vi "Write Integer Result to Log.vi"(7 "Test Class in":refnum<class "Test Class.lvclass">, 8 "error in (no error)":errorcluster, 9 "Label":string, 10 "Position":u32, 11 "Value":i64) -> (0 "error out":errorcluster)   [LabVIEW 2017, in "Test Class.lvclass"]
uses:
  Test Class.lvclass
  <vilib>/TSS/ACRObat Test Framework/Core Launcher/Core Manager Methods -- Enum.ctl
  <vilib>/TSS/ACRObat Test Framework/Classes/Data/Data Repo/Class/Data Repo.lvclass
  <vilib>/TSS/ACRObat Test Framework/Core Launcher/Core Launcher.lvlib
  Classes/Application/Class/Application.lvclass
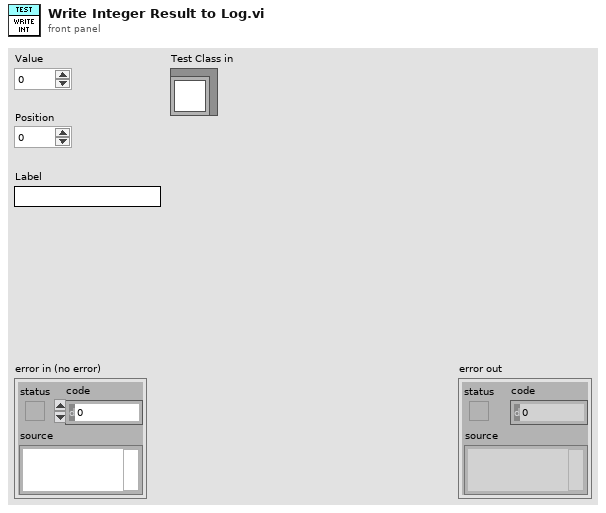
[diagram p1: front panel]
types:
  T1 = typedef "Core Launcher.lvlib/Core Manager Methods -- Enum.ctl" = enum16{"Spawn Objects", "Get Objects", "Destroy Objects"}
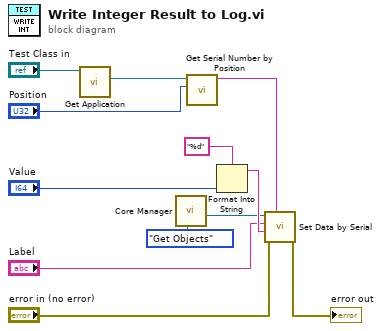
[diagram p0: block diagram]
diagram:
  n1 = call "Get Application.vi"("Test Class in"="Test Class in") -> ("Application.lvlib:Application.lvclass"=w7:refnum<class "Application.lvclass">)  [unwired: 9 in, 1 out]
  n2 = call <vilib>:"Core Manager.vi"("Method"=Core_Manager_Methods_--_Enum."Get Objects") -> ("Data Repo"=w9:refnum<class "Data Repo.lvclass">)  [unwired: 6 in, 4 out]
  n3 = call "Get Serial Number by Position.vi"("Position"="Position", "Application.lvclass"=w7) -> ("Value"=w11:string)  [unwired: 9 in]
  n4 = Format Into String(format string="%d", "Value") -> (resulting string=w10:string)  [unwired: 2 in, 1 out]
  n5 = call <vilib>:"Set Data by Serial.vi"("Serial"=w11, "error in (no error)"="error in (no error)", "Value"=w10, "Header"="Label", "Acrobat Template in"=w9) -> ("error out"=→"error out":errorcluster)  [unwired: 5 in, 1 out]
